vi "Delete Int8 DVR.vi"(8 "error in (no error)":errorcluster, 11 "Int8 DVR in":refnum<data-value>) -> (0 "error out":errorcluster, 3 "Int8 out":refnum<class "Int8.lvclass">)   [LabVIEW 2015, in "MDSplus.lvlib" / "Int8.lvclass"]
uses:
  Int8.lvclass
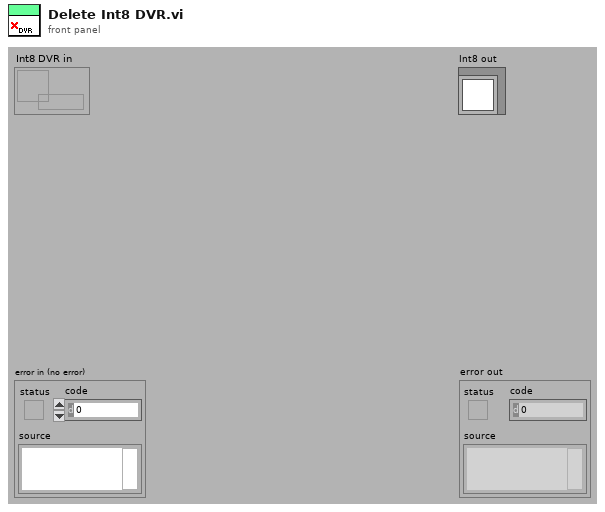
[diagram p1: front panel]
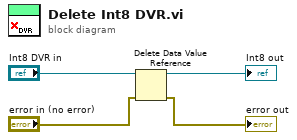
[diagram p0: block diagram]
diagram:
  n1 = Delete Data Value Reference(data value reference="Int8 DVR in", error in="error in (no error)") -> (data value=→"Int8 out":refnum<class "Int8.lvclass">, error out=→"error out":errorcluster)
